vi "Write devicesListCommand.vi"(8 "error in (no error)":errorcluster, 10 "devicesListCommand":string="$.list", 11 "SCD in":refnum<class "SCD.lvclass">) -> (0 "error out":errorcluster, 3 "SCD out":refnum<class "SCD.lvclass">)   [LabVIEW 2023, in "horiba.lvlib" / "SCD.lvclass"]
uses:
  SCD.lvclass
  SCD.lvclass/SCD.ctl
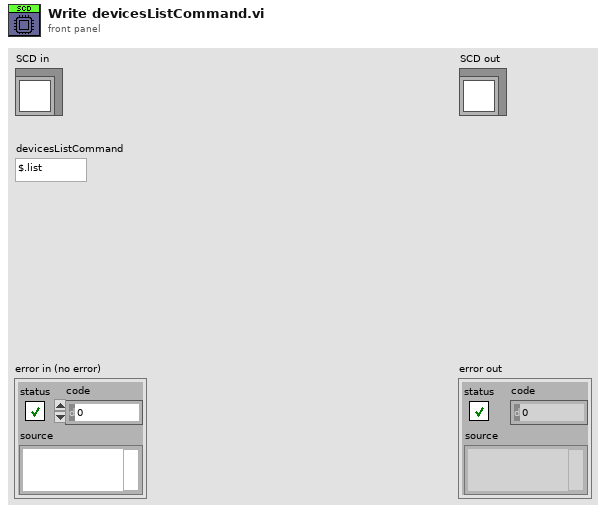
[diagram p1: front panel]
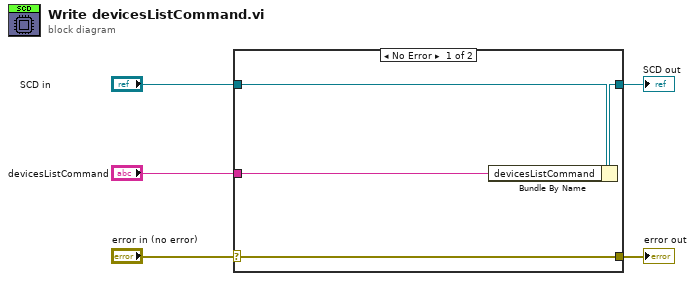
[diagram p0: block diagram]
diagram:
  n1 = case shown="No Error" "error in (no error)" {
    selector: "error in (no error)" -> [w9 w10]
    tunnel: [w9 w10] -> w4
    tunnel: [w7 w11] -> w2
    tunnel: "SCD in" -> [w8 w11]
    tunnel: "devicesListCommand" -> [w6 _]
    frame No Error {
      n2 = Bundle By Name(cluster=w8, "devicesListCommand"=w6) -> (w7:refnum<class "SCD.lvclass">)
    }
    frame Error {
    }
  }
  "error out" <- w4
  "SCD out" <- w2
